vi "CTRE_CANifier_ConfigSettings.vi"(6 "timeoutMs":i32=50, 7 "Force Write":bool, 8 "error in (no error)":errorcluster, 10 "CANifier Configuration":T1={"velocityMeasurementPeriod"=100, "velocityMeasurementWindow"=64, "clearPositionOnLimitF"=FALSE, "clearPositionOnLimitR"=FALSE, "clearPositionOnLimitQuadIdx"=FALSE, "CustomParam"={"customParam0"=0, "customParam1"=0}} {"velocityMeasurementPeriod" items=["Period_1Ms"=1, "Period_2Ms"=2, "Period_5Ms"=5, "Period_10Ms"=10, "Period_20Ms"=20, "Period_25Ms"=25, "Period_50Ms"=50, "Period_100Ms"=100]}, 11 "CANifierDevRef":T3) -> (0 "error out":errorcluster, 3 "CANifierDevRef":T3)   [LabVIEW 2020]
doc: "Configures all persistant settings\n\n<b> CANifier Configuration </b> Cluster of all the settings CANifier can be configured with"
uses:
  <vilib>/Rock Robotics/WPI/ThirdParty/Phoenix-LabVIEW/CANifier/CTRE_CANifier_DeviceRef.ctl
  <vilib>/Rock Robotics/WPI/ThirdParty/Phoenix-LabVIEW/CANifier/CTRE_CANifier_Configurables.ctl
  <vilib>/Rock Robotics/WPI/ThirdParty/Phoenix-LabVIEW/Controls/CTRE_Phoenix_CustomParamConfiguration.ctl
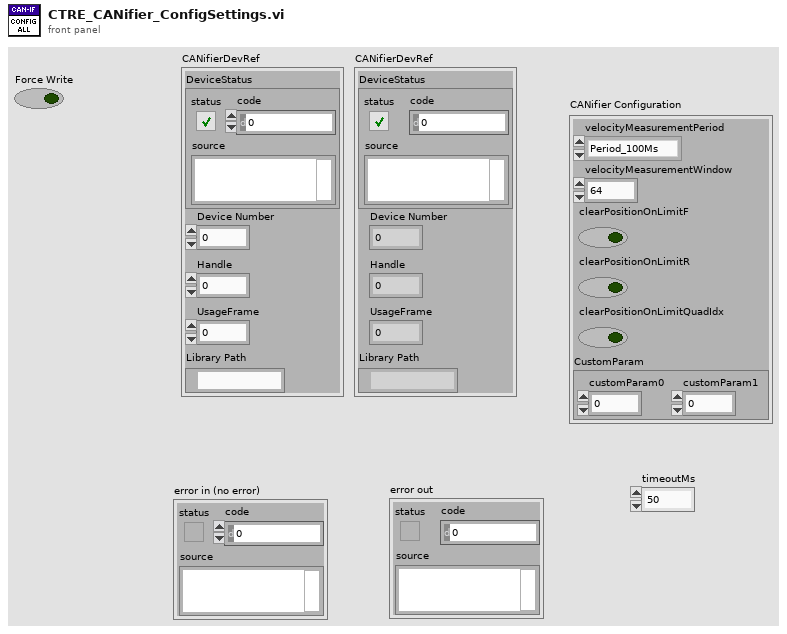
[diagram p1: front panel]
types:
  T1 = typedef "CTRE_CANifier_Configurables.ctl" = cluster{"velocityMeasurementPeriod":u16, "velocityMeasurementWindow":i32, "clearPositionOnLimitF":bool, "clearPositionOnLimitR":bool, "clearPositionOnLimitQuadIdx":bool, "CustomParam":T2}
  T2 = typedef "CTRE_Phoenix_CustomParamConfiguration.ctl" = cluster{"customParam0":i32, "customParam1":i32}
  T3 = typedef "CTRE_CANifier_DeviceRef.ctl" = cluster{"DeviceStatus":errorcluster, "Device Number":u8, "Handle":u64, "UsageFrame":u32, "Library Path":path}
  T4 = cluster{"velocityMeasurementPeriod":bool, "velocityMeasurementWindow":bool, "clearPositionOnLimitF":bool, "clearPositionOnLimitR":bool, "clearPositionOnLimitQuadIdx":bool, "CustomParam":cluster{"customParam0":bool, "customParam1":bool}}
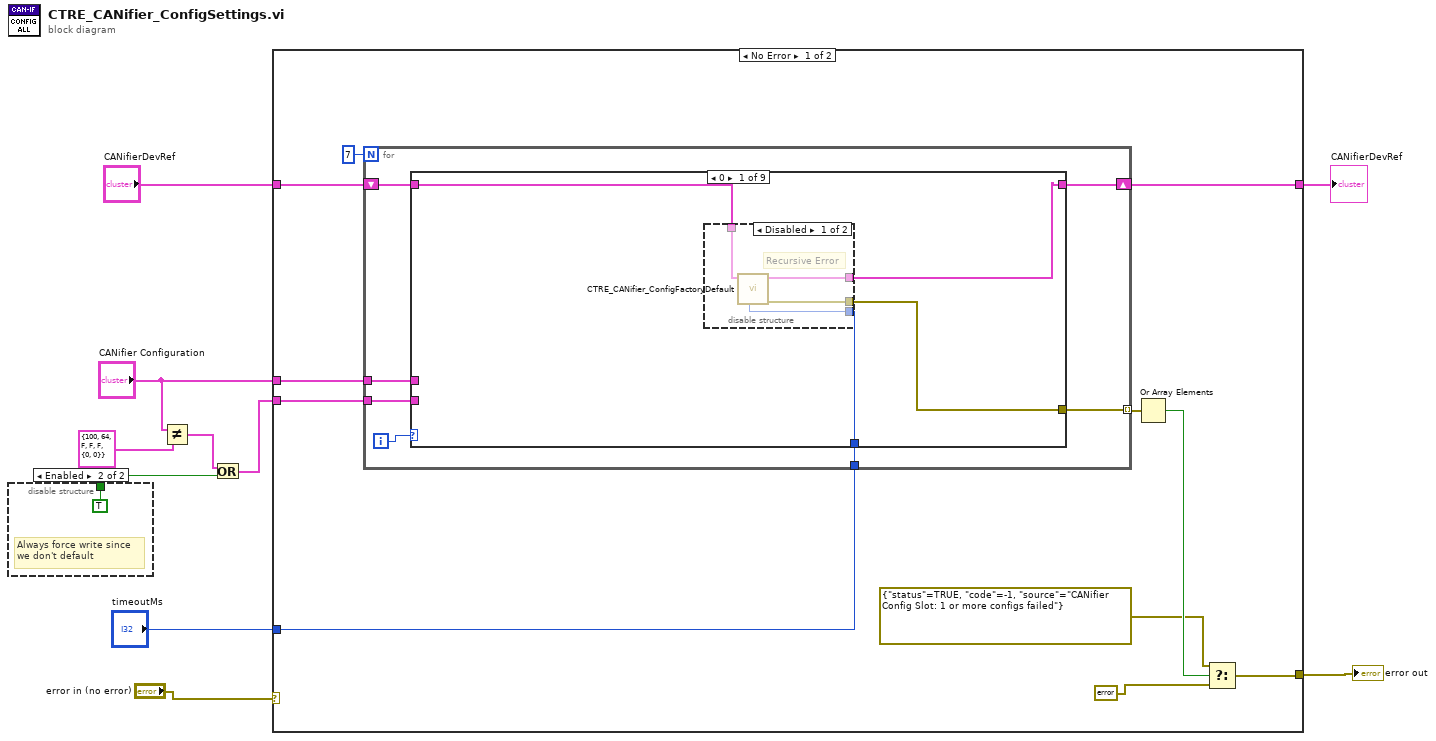
[diagram p0: block diagram]
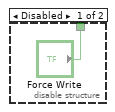
[diagram p2: hidden frame]
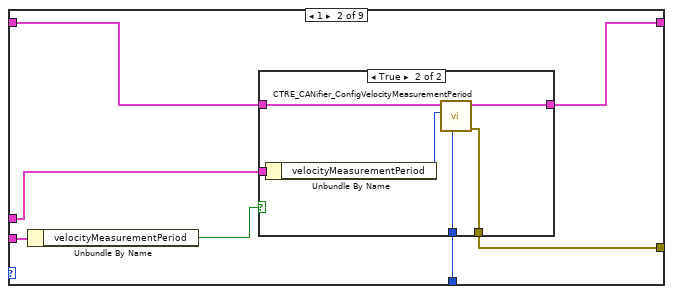
[diagram p4: hidden frame]
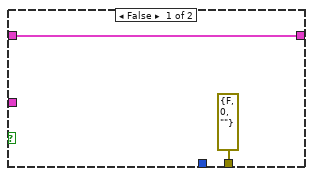
[diagram p5: hidden frame]
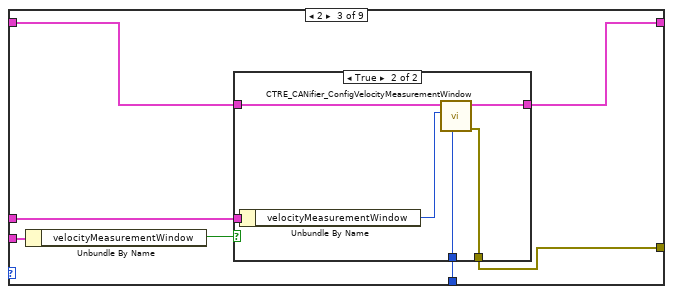
[diagram p6: hidden frame]
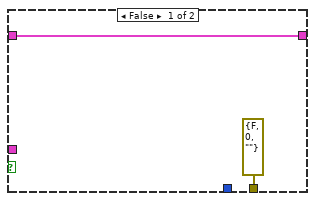
[diagram p7: hidden frame]
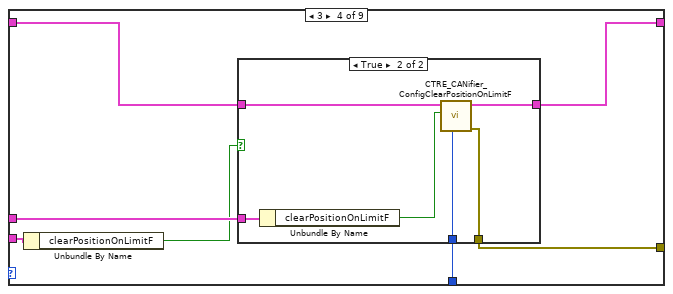
[diagram p8: hidden frame]
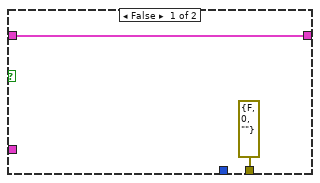
[diagram p9: hidden frame]
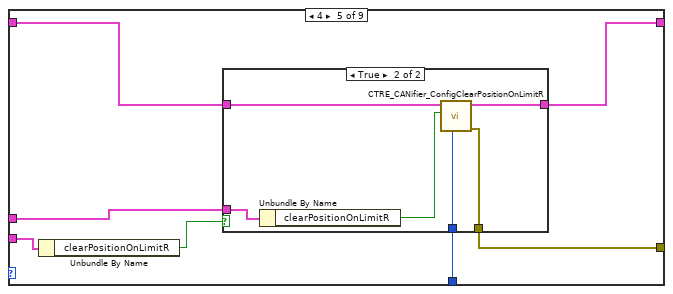
[diagram p10: hidden frame]
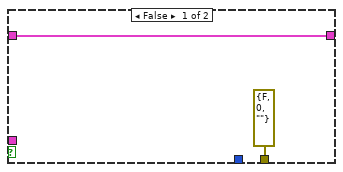
[diagram p11: hidden frame]
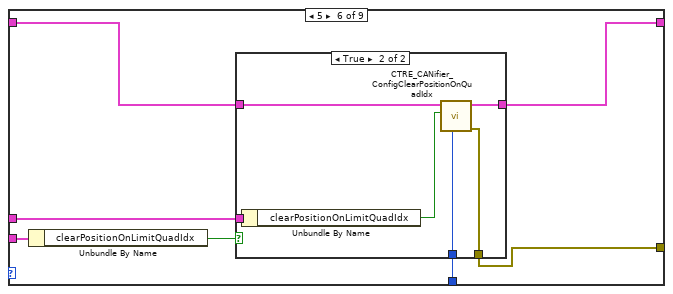
[diagram p12: hidden frame]
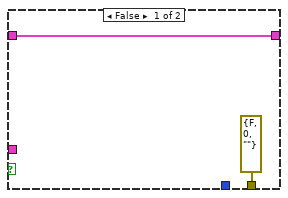
[diagram p13: hidden frame]
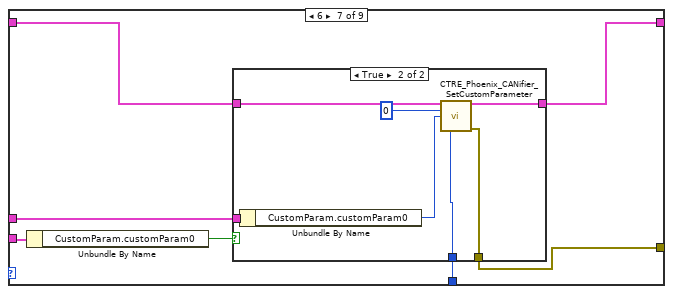
[diagram p14: hidden frame]
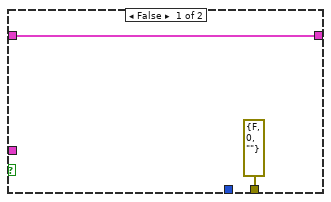
[diagram p15: hidden frame]
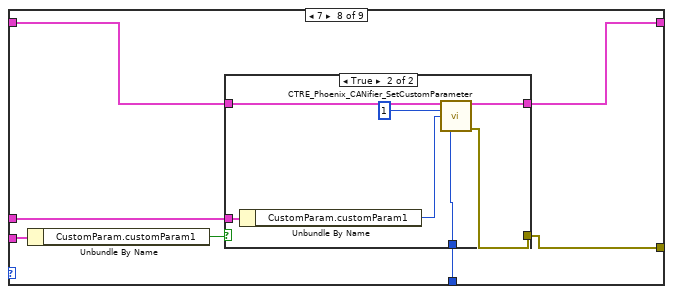
[diagram p16: hidden frame]
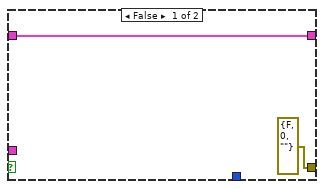
[diagram p17: hidden frame]
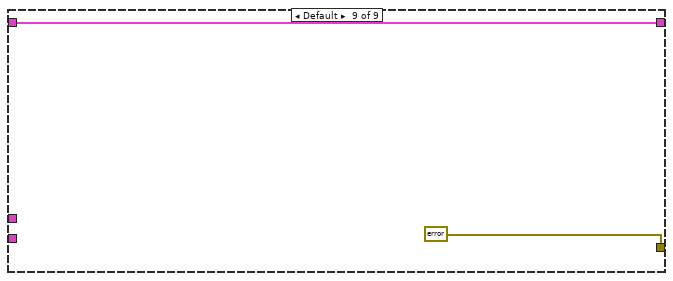
[diagram p18: hidden frame]
diagram:
  n1 = disable-structure shown="Enabled" {
    disable-tunnel: ["Force Write" TRUE ("Force Write")] -> w1
    frame Disabled {
    }
    frame Enabled {
      # "Always force write since\nwe don't default"
    }
  }
  n2 = Not Equal?(x="CANifier Configuration", y=T1 {"velocityMeasurementPeriod"=100, "velocityMeasurementWindow"=64, "clearPositionOnLimitF"=FALSE, "clearPositionOnLimitR"=FALSE, "clearPositionOnLimitQuadIdx"=FALSE, "CustomParam"={"customParam0"=0, "customParam1"=0}}) -> (x != y?=w3:T4)
  n3 = Or(x=w3, y=w1) -> (x .or. y?=w2:T4)
  n4 = case shown="No Error" "error in (no error)" {
    selector: "error in (no error)" -> [_ w150]
    tunnel: "CANifier Configuration" -> [w21 _]
    tunnel: "CANifierDevRef" -> [w23 w149]
    tunnel: [w22 w149] -> w8
    tunnel: "timeoutMs" -> [w20 _]
    tunnel: [w17 w150] -> w6
    tunnel: w2 -> [w13 _]
    frame No Error {
      n5 = for {
        N: 7 -> [_]
        shift-right: [w27] -> w22
        shift-left: w23 -> [w28]
        tunnel: w21 -> [w29]
        tunnel: w20 -> [w26]
        tunnel: [w25] -> w18 mode=indexing
        tunnel: w13 -> [w24]
        i -> [w30]
        n6 = case shown="0" w30 {
          tunnel: w29 -> [_ w42 w61 w76 w91 w106 w121 w137 _]
          tunnel: w28 -> [w34 w46 w60 w75 w90 w105 w120 w136 w148]
          tunnel: [w33 w45 w59 w74 w89 w104 w119 w135 w148] -> w27
          tunnel: w26 -> [w32 w44 w58 w73 w88 w103 w118 w134 _]
          tunnel: [w31 w43 w57 w72 w87 w102 w117 w133 errorcluster {"status"=FALSE, "code"=0, "source"=""} ("error out")] -> w25
          tunnel: w24 -> [_ w41 w56 w71 w86 w101 w116 w132 _]
          frame 0 {
            n7 = disable-structure shown="Disabled" {
              disable-tunnel: w34 -> [w38 w39]
              disable-tunnel: [w37 w39] -> w33
              disable-tunnel: w32 -> [w36 _]
              disable-tunnel: [w35 _] -> w31
              frame Disabled {
                # "Recursive Error"
                n8 = call <vilib>:"CTRE_CANifier_ConfigFactoryDefault.vi"("timeoutMs"=w36, "CANifierDevRef"=w38) -> ("error out"=w35:errorcluster, "CANifierDevRef"=w37:T3)  [unwired: 8 in]
              }
              frame Enabled {
              }
            }
          }
          frame 1 {
            n9 = Unbundle By Name(w41) -> ("velocityMeasurementPeriod"=w40:bool)
            n10 = case shown="True" w40 {
              tunnel: w46 -> [w48 w54]
              tunnel: [w48 w53] -> w45
              tunnel: w44 -> [_ w51]
              tunnel: [errorcluster {"status"=FALSE, "code"=0, "source"=""} ("error out") w50] -> w43
              tunnel: w42 -> [_ w49]
              frame False {
              }
              frame True {
                n11 = Unbundle By Name(w49) -> ("velocityMeasurementPeriod"=w52:u16)
                n12 = call <vilib>:"CTRE_CANifier_ConfigVelocityMeasurementPeriod.vi"("timeoutMs"=w51, "Period"=w52, "CANifierDevRef"=w54) -> ("error out"=w50:errorcluster, "CANifierDevRef"=w53:T3)  [unwired: 7 in]
              }
            }
          }
          frame 2 {
            n13 = Unbundle By Name(w56) -> ("velocityMeasurementWindow"=w55:bool)
            n14 = case shown="True" w55 {
              tunnel: w61 -> [_ w69]
              tunnel: w60 -> [w63 w68]
              tunnel: [w63 w67] -> w59
              tunnel: w58 -> [_ w65]
              tunnel: [errorcluster {"status"=FALSE, "code"=0, "source"=""} ("error out") w64] -> w57
              frame False {
              }
              frame True {
                n15 = Unbundle By Name(w69) -> ("velocityMeasurementWindow"=w66:i32)
                n16 = call <vilib>:"CTRE_CANifier_ConfigVelocityMeasurementWindow.vi"("timeoutMs"=w65, "windowSize"=w66, "CANifierDevRef"=w68) -> ("error out"=w64:errorcluster, "CANifierDevRef"=w67:T3)  [unwired: 7 in]
              }
            }
          }
          frame 3 {
            n17 = Unbundle By Name(w71) -> ("clearPositionOnLimitF"=w70:bool)
            n18 = case shown="True" w70 {
              tunnel: w76 -> [_ w84]
              tunnel: w75 -> [w78 w83]
              tunnel: [w78 w82] -> w74
              tunnel: w73 -> [_ w81]
              tunnel: [errorcluster {"status"=FALSE, "code"=0, "source"=""} ("error out") w79] -> w72
              frame False {
              }
              frame True {
                n19 = Unbundle By Name(w84) -> ("clearPositionOnLimitF"=w80:bool)
                n20 = call <vilib>:"CTRE_CANifier_ConfigClearPositionOnLimitF.vi"("timeoutMs"=w81, "clearPositionOnLimitF"=w80, "CANifierDevRef"=w83) -> ("error out"=w79:errorcluster, "CANifierDevRef"=w82:T3)  [unwired: 7 in]
              }
            }
          }
          frame 4 {
            n21 = Unbundle By Name(w86) -> ("clearPositionOnLimitR"=w85:bool)
            n22 = case shown="True" w85 {
              tunnel: w91 -> [_ w99]
              tunnel: w90 -> [w93 w98]
              tunnel: [w93 w97] -> w89
              tunnel: w88 -> [_ w96]
              tunnel: [errorcluster {"status"=FALSE, "code"=0, "source"=""} ("error out") w94] -> w87
              frame False {
              }
              frame True {
                n23 = Unbundle By Name(w99) -> ("clearPositionOnLimitR"=w95:bool)
                n24 = call <vilib>:"CTRE_CANifier_ConfigClearPositionOnLimitR.vi"("timeoutMs"=w96, "clearPositionOnLimitR"=w95, "CANifierDevRef"=w98) -> ("error out"=w94:errorcluster, "CANifierDevRef"=w97:T3)  [unwired: 7 in]
              }
            }
          }
          frame 5 {
            n25 = Unbundle By Name(w101) -> ("clearPositionOnLimitQuadIdx"=w100:bool)
            n26 = case shown="True" w100 {
              tunnel: w106 -> [_ w114]
              tunnel: w105 -> [w108 w113]
              tunnel: [w108 w112] -> w104
              tunnel: w103 -> [_ w111]
              tunnel: [errorcluster {"status"=FALSE, "code"=0, "source"=""} ("error out") w109] -> w102
              frame False {
              }
              frame True {
                n27 = Unbundle By Name(w114) -> ("clearPositionOnLimitQuadIdx"=w110:bool)
                n28 = call <vilib>:"CTRE_CANifier_ConfigClearPositionOnQuadIdx.vi"("timeoutMs"=w111, "clearPositionOnQuadIdx"=w110, "CANifierDevRef"=w113) -> ("error out"=w109:errorcluster, "CANifierDevRef"=w112:T3)  [unwired: 7 in]
              }
            }
          }
          frame 6 {
            n29 = Unbundle By Name(w116) -> ("CustomParam.customParam0"=w115:bool)
            n30 = case shown="True" w115 {
              tunnel: w121 -> [_ w130]
              tunnel: w120 -> [w123 w129]
              tunnel: [w123 w128] -> w119
              tunnel: w118 -> [_ w127]
              tunnel: [errorcluster {"status"=FALSE, "code"=0, "source"=""} ("error out") w126] -> w117
              frame False {
              }
              frame True {
                n31 = Unbundle By Name(w130) -> ("CustomParam.customParam0"=w125:i32)
                n32 = call <vilib>:"CTRE_Phoenix_CANifier_SetCustomParameter.vi"("CTRE_CANifier_DeviceRef"=w129, "paramIdx"=u32 0, "value"=w125, "timeoutMs"=w127) -> ("CTRE_CANifier_DeviceRef"=w128:T3, "error out"=w126:errorcluster)  [unwired: 10 in]
              }
            }
          }
          frame 7 {
            n33 = Unbundle By Name(w132) -> ("CustomParam.customParam1"=w131:bool)
            n34 = case shown="True" w131 {
              tunnel: w137 -> [_ w146]
              tunnel: w136 -> [w139 w145]
              tunnel: [w139 w144] -> w135
              tunnel: w134 -> [_ w143]
              tunnel: [errorcluster {"status"=FALSE, "code"=0, "source"=""} ("error out") w142] -> w133
              frame False {
              }
              frame True {
                n35 = Unbundle By Name(w146) -> ("CustomParam.customParam1"=w141:i32)
                n36 = call <vilib>:"CTRE_Phoenix_CANifier_SetCustomParameter.vi"("CTRE_CANifier_DeviceRef"=w145, "paramIdx"=u32 1, "value"=w141, "timeoutMs"=w143) -> ("CTRE_CANifier_DeviceRef"=w144:T3, "error out"=w142:errorcluster)  [unwired: 10 in]
              }
            }
          }
          frame Default {
          }
        }
      }
      n37 = Or Array Elements(Boolean array=w18) -> (logical OR=w16:bool)
      n38 = Select(t=errorcluster {"status"=TRUE, "code"=-1, "source"="CANifier Config Slot: 1 or more configs failed"} ("error out"), s=w16, f=errorcluster {"status"=FALSE, "code"=0, "source"=""} ("error out")) -> (s? t:f=w17:errorcluster)
    }
    frame Error {
    }
  }
  "CANifierDevRef" <- w8
  "error out" <- w6
